vi "test Import Same Module Different Configuration.vi"(8 "error in (no error)":errorcluster, 11 "TestCase in":refnum<class "SLSC Switch Import Export Unit Tests.lvclass">) -> (0 "error out":errorcluster, 3 "TestCase out":refnum<class "SLSC Switch Import Export Unit Tests.lvclass">)   [LabVIEW 2017, in "SLSC Switch Import Export Unit Tests.lvclass"]
uses:
  SLSC Switch Import Export Unit Tests.lvclass
  Shared/Endpoint Configuration Cluster.ctl
  Shared/Endpoint Configuration Enum.ctl
  SLSC Switch Import Export Unit Tests.lvclass/SLSC Switch Import Export Unit Tests.ctl
  <vilib>/addons/_JKI Toolkits/VI Tester/TestCase.llb/TestCase.lvclass
  <vilib>/NI/NI VeriStand Custom Device Import and Export Tool/ImportExport.lvlib
  Scripting/SLSC Switch Scripting.lvlib
  Shared/VeriStand System Definition Test Utilities/VeriStand System Definition Test Utilities.lvlib
  Shared/SLSC Switch Shared.lvlib
  C:/Program Files (x86)/National Instruments/LabVIEW 2017/vi.lib/addons/_JKI Toolkits/VI Tester/TestCase.llb/TestCase.lvclass
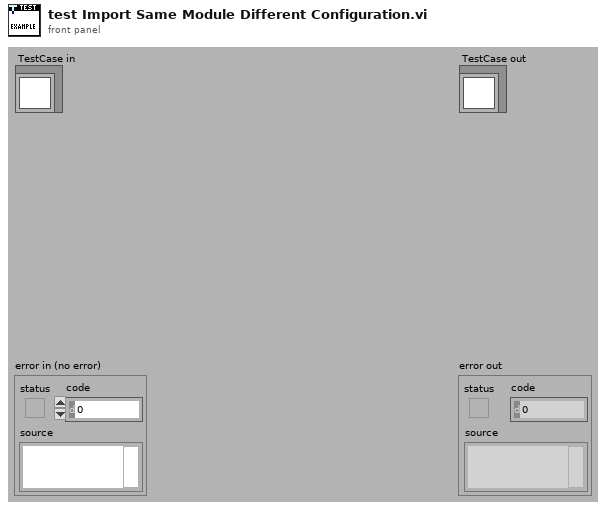
[diagram p1: front panel]
types:
  T1 = typedef "SLSC Switch Shared.lvlib/Endpoint Configuration Cluster.ctl" = cluster{"Endpoint":string, "Configuration":T2}
  T2 = typedef "SLSC Switch Shared.lvlib/Endpoint Configuration Enum.ctl" = enum16{"Load", "Source", "Configuration"}
  T3 = cluster{"Ignore Properties":string[], "Ignore Top Level Name":bool}
  T4 = typedef "Custom Device API.lvlib/Custom Device Item Ref.ctl" = u64
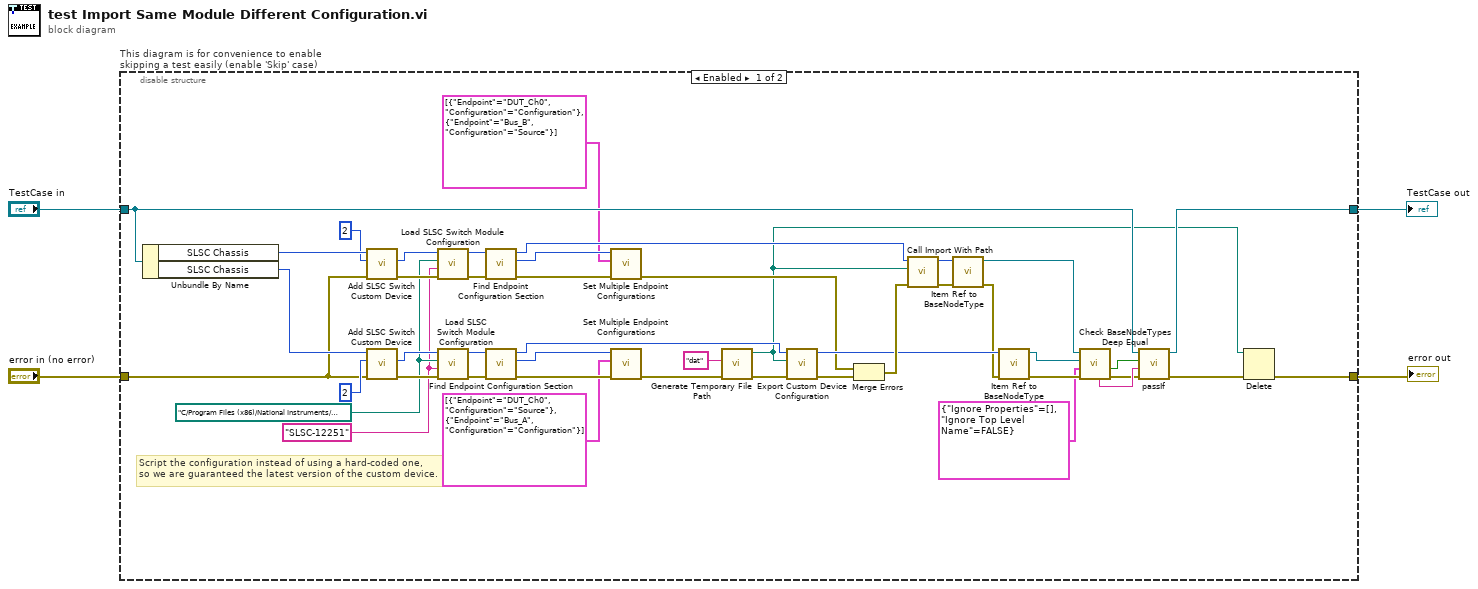
[diagram p0: block diagram]
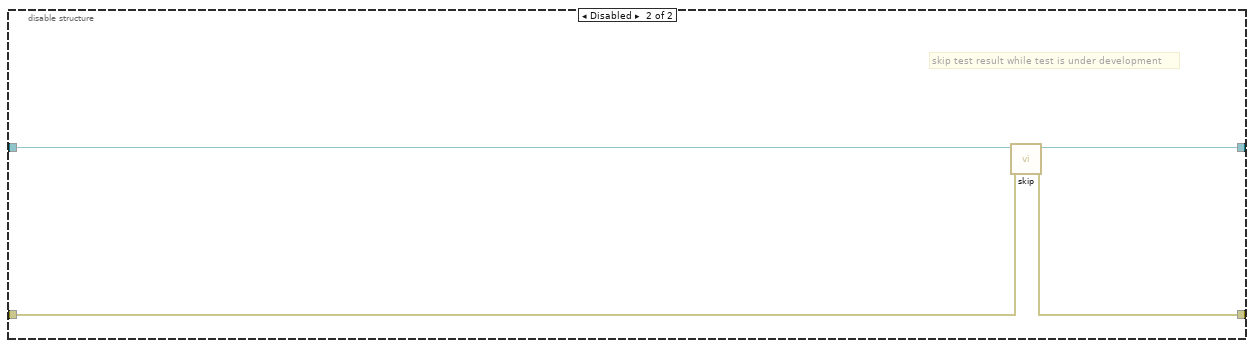
[diagram p2: hidden frame]
diagram:
  n1 = disable-structure "This diagram is for convenience to enable skipping a test easily (enable 'Skip' case)" shown="Enabled" {
    disable-tunnel: "TestCase in" -> [w37 w53]
    disable-tunnel: [w8 w51] -> w1
    disable-tunnel: [w6 w52] -> w3
    disable-tunnel: "error in (no error)" -> [w31 w50]
    frame Enabled {
      w17 = path "C:/Program Files (x86)/National Instruments/Shared/NI-SLSC Switch/Modules/SLSC-12251-switches.json" ("switches json file")
      w16 = "SLSC-12251" ("product name")
      # "Script the configuration instead of using a hard-coded one,\nso we are guaranteed the latest version of the custom device."
      n2 = Unbundle By Name(w37) -> ("SLSC Chassis"=w32:u64, "SLSC Chassis"=w49:u64)
      n3 = call "Add SLSC Switch Custom Device.vi"("error in"=w31, "slot number"=u32 2, "slsc chassis in"=w32) -> ("error out"=w19:errorcluster, "slsc switch custom device"=w15:T4)  [unwired: 6 in, 1 out]
      n4 = call "Add SLSC Switch Custom Device.vi"("error in"=w31, "slot number"=u32 2, "slsc chassis in"=w49) -> ("error out"=w30:errorcluster, "slsc switch custom device"=w28:T4)  [unwired: 6 in, 1 out]
      n5 = call "Load SLSC Switch Module Configuration.vi"("error in"=w19, "product name"=w16, "switches json file"=w17, "slsc switch custom device in"=w15) -> ("error out"=w18:errorcluster, "slsc switch custom device out"=w20:T4)  [unwired: 6 in]
      n6 = call "Load SLSC Switch Module Configuration.vi"("error in"=w30, "product name"=w16, "switches json file"=w17, "slsc switch custom device in"=w28) -> ("error out"=w29:errorcluster, "slsc switch custom device out"=w26:T4)  [unwired: 6 in]
      n7 = call "Find Endpoint Configuration Section.vi"("error in"=w18, "slsc switch custom device in"=w20) -> ("error out"=w14:errorcluster, "endpoint configuration"=w12:T4, "slsc switch custom device out"=w11:T4)  [unwired: 7 in]
      n8 = call "Find Endpoint Configuration Section.vi"("error in"=w29, "slsc switch custom device in"=w26) -> ("error out"=w27:errorcluster, "endpoint configuration"=w24:T4, "slsc switch custom device out"=w23:T4)  [unwired: 7 in]
      n9 = call "Set Multiple Endpoint Configurations.vi"("error in"=w14, "endpoint configurations"=T1[] [{"Endpoint"="DUT_Ch0", "Configuration"=enum."Configuration"}, {"Endpoint"="Bus_B", "Configuration"=enum."Source"}], "endpoint configuration in"=w12) -> ("error out"=w10:errorcluster)  [unwired: 7 in, 1 out]
      n10 = call "Set Multiple Endpoint Configurations.vi"("error in"=w27, "endpoint configurations"=T1[] [{"Endpoint"="DUT_Ch0", "Configuration"=enum."Source"}, {"Endpoint"="Bus_A", "Configuration"=enum."Configuration"}], "endpoint configuration in"=w24) -> ("error out"=w25:errorcluster)  [unwired: 7 in, 1 out]
      n11 = call <vilib>:"Generate Temporary File Path.vi"("error in (no error)"=w25, "Temporary File Extension (tmp)"="dat") -> ("error out"=w46:errorcluster, "Unique Temporary File Path"=w5:path)  [unwired: 8 in]
      n12 = call <vilib>:"Export Custom Device Configuration.vi"("error in (no error)"=w46, "Path"=w5, "ID"=w23) -> ("error out"=w45:errorcluster, "ID out"=w42:u64)  [unwired: 7 in]
      n13 = Merge Errors(w10, w45) -> (w44:errorcluster)
      n14 = call "Call Import With Path.vi"("error in (no error)"=w44, "Path"=w5, "Node Ptr"=w11) -> ("error out"=w41:errorcluster, "Node Ptr out"=w43:u64)  [unwired: 7 in]
      n15 = call "Item Ref to BaseNodeType.vi"("error in (no error)"=w41, "Item Ref"=w43) -> ("error out"=w40:errorcluster, "BaseNodeType"=w34:refnum<k24>)  [unwired: 8 in]
      n16 = call "Item Ref to BaseNodeType.vi"("error in (no error)"=w40, "Item Ref"=w42) -> ("error out"=w39:errorcluster, "BaseNodeType"=w38:refnum<k24>)  [unwired: 8 in]
      n17 = call "Check BaseNodeTypes Deep Equal.vi"("error in (no error)"=w39, "Settings"=T3 {"Ignore Properties"=[], "Ignore Top Level Name"=FALSE}, "BaseNodeType 2"=w38, "BaseNodeType 1"=w34) -> ("error out"=w33:errorcluster, "Equal?"=w36:bool, "Inequality context"=w35:string)  [unwired: 3 in, 2 out]
      n18 = call-dynamic "passIf.vi"("error in (no error)"=w33, "message (\"\")"=w35, "pass"=w36, "TestCase in"=w37) -> ("error out"=w7:errorcluster, "TestCase out"=w8:refnum<class "SLSC Switch Import Export Unit Tests.lvclass">)  [unwired: 6 in]
      n19 = Delete(path (use dialog)=w5, error in=w7) -> (error out=w6:errorcluster)  [unwired: 3 in, 2 out]
    }
    frame Disabled {
      # "skip test result while test is under development"
      n20 = call <vilib>:"skip.vi"("error in (no error)"=w50, "TestCase in"=w53) -> ("error out"=w52:errorcluster, "TestCase out"=w51:refnum<class "SLSC Switch Import Export Unit Tests.lvclass">)  [unwired: 8 in]
    }
  }
  "error out" <- w3
  "TestCase out" <- w1
